vi "Read Gates From Registry.vi"(7 "Micropulse No.":i32, 8 "error in (no error)":errorcluster, 11 "Test No.":u32) -> (0 "error out":errorcluster, 1 "Multi Gate Inspection":T3 {"Gate 4"."Max # Peaks" max=64000 step=100; "Gate 4"."Threshold" min=10 max=4095 step=10; "Gate 4"."Length (us)" min=0.0 max=96000.0 step=100.0; "Gate 4"."Start (us)" min=0.0 max=64000.0 step=100.0; "Gate 3"."Max # Peaks" max=64000 step=100; "Gate 3"."Threshold" min=10 max=4095 step=10; "Gate 3"."Length (us)" min=0.0 max=96000.0 step=100.0; "Gate 3"."Start (us)" min=0.0 max=64000.0 step=100.0; "Gate 2"."Max # Peaks" max=64000 step=100; "Gate 2"."Threshold" min=10 max=4095 step=10; "Gate 2"."Length (us)" min=0.0 max=96000.0 step=100.0; "Gate 2"."Start (us)" min=0.0 max=64000.0 step=100.0; "Gate 1"."Max # Peaks" max=64000 step=100; "Gate 1"."Threshold" min=10 max=4095 step=10; "Gate 1"."Length (us)" min=0.0 max=96000.0 step=100.0; "Gate 1"."Start (us)" min=0.0 max=64000.0 step=100.0}, 2 "Echo Gate Parameters":T2={"Start (us)"=0.0, "Length (us)"=0.0, "Threshold"=10} {"Threshold" min=10 max=4095 step=10; "Length (us)" min=0.0 max=96000.0 step=100.0; "Start (us)" min=0.0 max=64000.0 step=100.0}, 3 "Echo Gate Mode":T1)   [LabVIEW 2015]
uses:
  <instrlib>/Micropulse/Public/Data/Datatypes/MP - multi-gate inspection.ctl
  <instrlib>/Micropulse/Public/Data/Datatypes/MP - multigate inspection gate parameters.ctl
  <instrlib>/Micropulse/Public/Data/Datatypes/MP - hysteresis level.ctl
  <instrlib>/Micropulse/Public/Data/Datatypes/MP - multigate mode.ctl
  <instrlib>/Micropulse/Public/Data/Datatypes/MP - echo gate parameters.ctl
  <instrlib>/Micropulse/Public/Data/Datatypes/MP - echo gate mode.ctl
  <instrlib>/Micropulse/Micropulse.lvlib
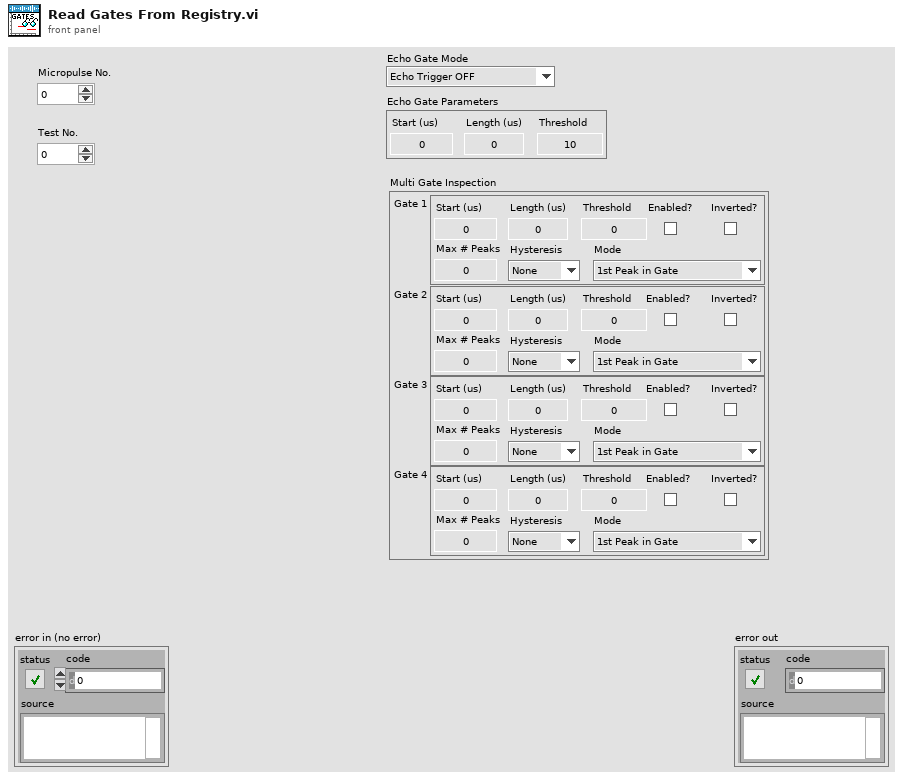
[diagram p1: front panel]
types:
  T1 = typedef "Micropulse.lvlib/MP - echo gate mode.ctl" = enum16{"Echo Trigger OFF", "Echo Gate Display Mode", "Echo Trigger ON", "Multi Gate or FMC Mode", "Reserved", "PA - Echo Trigger ON"}
  T2 = typedef "MP - echo gate parameters.ctl" = cluster{"Start (us)":dbl, "Length (us)":dbl, "Threshold":u16}
  T3 = typedef "MP - multi-gate inspection.ctl" = cluster{"Gate 1":T4, "Gate 2":T4, "Gate 3":T4, "Gate 4":T4}
  T4 = typedef "Micropulse.lvlib/MP - multigate inspection gate parameters.ctl" = cluster{"Start (us)":dbl, "Length (us)":dbl, "Threshold":u16, "Enabled?":bool, "Max # Peaks":u16, "Hysteresis":T5, "Mode":T6, "Inverted?":bool}
  T5 = typedef "Micropulse.lvlib/MP - hysteresis level.ctl" = enum16{"None", "3dB", "6dB", "9dB", "12dB"}
  T6 = typedef "Micropulse.lvlib/MP - multigate mode.ctl" = enum16{"1st Peak in Gate", "Largest Peak In Gate", "All Peaks In Gate", "1st Threshold Crossing"}
  T7 = typedef "Micropulse.lvlib/MP-Registry Data-Cluster.ctl" = cluster{"Instrument Type":T8, "Serial #":u64, "Sample Frequency":T9, "dt (us)":dbl, "DOF":T10, "Material Velocity":dbl, "Asynch Reads":T11, "NUM of Tests":u16, "Gates":T12[], "CMD LUT":variant, "Command List":string}
  T8 = typedef "Micropulse.lvlib/MP - instrument type.ctl" = enum16{"MicroPulse 5", "MicroPulse LT1", "MicroPulse LT2", "MicroPulse LTPA", "MPLT", "MicroPulse 6", "<MicroPulse>", "Simulated Data"}
  T9 = typedef "Micropulse.lvlib/MP - sample frequency.ctl" = enum16{"Use Default", "200MHz (LT2 only)", "100MHz", "50MHz", "25MHz", "10MHz"}
  T10 = typedef "Micropulse.lvlib/MP - data output format.ctl" = enum16{"", "8-bit Mode", "10-bit Mode", "12-bit Mode", "16-bit Mode", "8-bit Log Mode", "12-bit Packed Mode"}
  T11 = typedef "Micropulse.lvlib/MP - asynch read mode.ctl" = enum16{"Disabled", "Enabled"}
  T12 = typedef "Micropulse.lvlib/MP - Registry Gates.ctl" = cluster{"Display Gate":T13, "ETM Mode":T1, "Echo Gate":T2, "Insp Gates":T4[]}
  T13 = typedef "MP - display gate.ctl" = cluster{"Start":dbl, "Length":dbl}
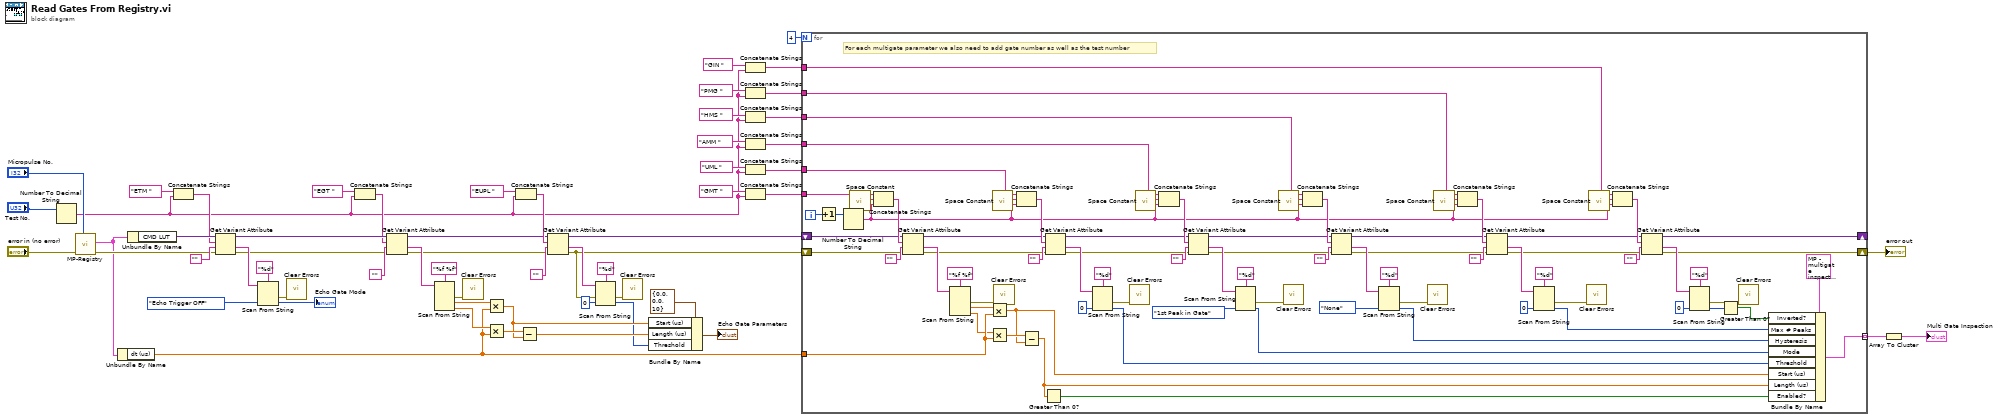
[diagram p0: block diagram]
diagram:
  n1 = Number To Decimal String(number="Test No.") -> (decimal integer string=w12:string)  [unwired: 1 in]
  n2 = call <instrlib>:"MP-Registry.vi"("Micropulse # In"="Micropulse No.", "error in (no error)"="error in (no error)") -> ("error out"=w54:errorcluster, "Micropulse Data"=w35:T7)  [unwired: 6 in, 2 out]
  n3 = Unbundle By Name(w35) -> ("dt (us)"=w20:dbl)
  n4 = Unbundle By Name(w35) -> ("CMD LUT"=w57:variant)
  n5 = Concatenate Strings("ETM " ("name"), w12) -> (w46:string)
  n6 = Get Variant Attribute(Variant=w57, name=w46, default value (empty Variant)="", error in=w54) -> (duplicate Variant=w49:variant, value=w53:string, error out=w4:errorcluster)  [unwired: 1 out]
  n7 = Scan From String(format string="%d", input string=w53, default 1=MP_-_echo_gate_mode."Echo Trigger OFF" ("Echo Gate Mode")) -> (error out=w2:errorcluster, output 1=→"Echo Gate Mode":T1)  [unwired: 2 in, 2 out]
  n8 = call <vilib>:"Clear Errors.vi"("error in (no error)"=w2) -> ()  [unwired: 5 in, 2 out]
  n9 = Concatenate Strings("EGT " ("name"), w12) -> (w44:string)
  n10 = Get Variant Attribute(Variant=w49, name=w44, default value (empty Variant)="", error in=w4) -> (duplicate Variant=w27:variant, value=w42:string, error out=w5:errorcluster)  [unwired: 1 out]
  n11 = Scan From String(format string="%f %f", input string=w42) -> (error out=w1:errorcluster, output 1=w34:dbl, output 2=w33:dbl)  [unwired: 4 in, 2 out]
  n12 = call <vilib>:"Clear Errors.vi"("error in (no error)"=w1) -> ()  [unwired: 5 in, 2 out]
  n13 = Multiply(x=w34, y=w20) -> (x*y=w29:dbl)
  n14 = Multiply(x=w33, y=w20) -> (x*y=w32:dbl)
  n15 = Concatenate Strings("EUPL " ("name"), w12) -> (w39:string)
  n16 = Subtract(x=w32, y=w29) -> (x-y=w30:dbl)
  n17 = Get Variant Attribute(Variant=w27, name=w39, default value (empty Variant)="", error in=w5) -> (duplicate Variant=w22:variant, value=w41:string, error out=w3:errorcluster)  [unwired: 1 out]
  n18 = Scan From String(format string="%d", input string=w41, error in=w3, default 1=u16 0 ("default value 1")) -> (error out=w21:errorcluster, output 1=w28:u16)  [unwired: 1 in, 2 out]
  n19 = call <vilib>:"Clear Errors.vi"("error in (no error)"=w21) -> ()  [unwired: 5 in, 2 out]
  n20 = Bundle By Name(cluster=T2 {"Start (us)"=0.0, "Length (us)"=0.0, "Threshold"=10} ("Echo Gate Parameters"), "Start (us)"=w29, "Length (us)"=w30, "Threshold"=w28) -> (→"Echo Gate Parameters":T2)
  n21 = Concatenate Strings("GIN " ("name"), w12) -> (w9:string)
  n22 = Concatenate Strings("PMG " ("name"), w12) -> (w10:string)
  n23 = Concatenate Strings("HMS " ("name"), w12) -> (w11:string)
  n24 = Concatenate Strings("AMM " ("name"), w12) -> (w16:string)
  n25 = Concatenate Strings("UML " ("name"), w12) -> (w18:string)
  n26 = Concatenate Strings("GMT " ("name"), w12) -> (w24:string)
  n27 = for {
    N: 4 -> [_]
    tunnel: w24 -> [w137]
    shift-right: [w88] -> _
    shift-left: w22 -> [w130]
    shift-right: [w69] -> w8
    shift-left: w3 -> [w129]
    tunnel: w20 -> [w126]
    tunnel: w18 -> [w119]
    tunnel: w16 -> [w111]
    tunnel: w11 -> [w86]
    tunnel: w10 -> [w85]
    tunnel: w9 -> [w84]
    tunnel: [w73] -> w7 mode=indexing
    i -> [w133]
    # "For each multigate parameter we also need to add gate number as well as the test number"
    n28 = Increment(x=w133) -> (x+1=w132:i32)
    n29 = Number To Decimal String(number=w132) -> (decimal integer string=w72:string)  [unwired: 1 in]
    n30 = call <vilib>:"Space Constant.vi"() -> ("String"=w131:string)
    n31 = Concatenate Strings(w137, w131, w72) -> (w134:string)
    n32 = Get Variant Attribute(Variant=w130, name=w134, default value (empty Variant)="", error in=w129) -> (duplicate Variant=w118:variant, value=w135:string, error out=w71:errorcluster)  [unwired: 1 out]
    n33 = Scan From String(format string="%f %f", input string=w135) -> (error out=w70:errorcluster, output 1=w127:dbl, output 2=w125:dbl)  [unwired: 4 in, 2 out]
    n34 = Multiply(x=w127, y=w126) -> (x*y=w74:dbl)
    n35 = Multiply(x=w125, y=w126) -> (x*y=w128:dbl)
    n36 = call <vilib>:"Space Constant.vi"() -> ("String"=w124:string)
    n37 = call <vilib>:"Clear Errors.vi"("error in (no error)"=w70) -> ()  [unwired: 5 in, 2 out]
    n38 = Concatenate Strings(w119, w124, w72) -> (w120:string)
    n39 = Subtract(x=w128, y=w74) -> (x-y=w75:dbl)
    n40 = Greater Than 0?(x=w75) -> (x > 0?=w76:bool)
    n41 = Get Variant Attribute(Variant=w118, name=w120, default value (empty Variant)="", error in=w71) -> (duplicate Variant=w109:variant, value=w123:string, error out=w61:errorcluster)  [unwired: 1 out]
    n42 = Scan From String(format string="%d", input string=w123, default 1=u16 0 ("default value 1")) -> (error out=w60:errorcluster, output 1=w77:u16)  [unwired: 2 in, 2 out]
    n43 = call <vilib>:"Clear Errors.vi"("error in (no error)"=w60) -> ()  [unwired: 5 in, 2 out]
    n44 = call <vilib>:"Space Constant.vi"() -> ("String"=w112:string)
    n45 = Concatenate Strings(w111, w112, w72) -> (w116:string)
    n46 = Get Variant Attribute(Variant=w109, name=w116, default value (empty Variant)="", error in=w61) -> (duplicate Variant=w91:variant, value=w113:string, error out=w63:errorcluster)  [unwired: 1 out]
    n47 = Scan From String(format string="%d", input string=w113, default 1=MP_-_multigate_mode."1st Peak in Gate" ("Value")) -> (error out=w62:errorcluster, output 1=w78:T6)  [unwired: 2 in, 2 out]
    n48 = call <vilib>:"Space Constant.vi"() -> ("String"=w104:string)
    n49 = call <vilib>:"Clear Errors.vi"("error in (no error)"=w62) -> ()  [unwired: 5 in, 2 out]
    n50 = Concatenate Strings(w86, w104, w72) -> (w108:string)
    n51 = Get Variant Attribute(Variant=w91, name=w108, default value (empty Variant)="", error in=w63) -> (duplicate Variant=w90:variant, value=w105:string, error out=w65:errorcluster)  [unwired: 1 out]
    n52 = Scan From String(format string="%d", input string=w105, default 1=MP_-_hysteresis_level."None" ("Value")) -> (error out=w64:errorcluster, output 1=w79:T5)  [unwired: 2 in, 2 out]
    n53 = call <vilib>:"Clear Errors.vi"("error in (no error)"=w64) -> ()  [unwired: 5 in, 2 out]
    n54 = call <vilib>:"Space Constant.vi"() -> ("String"=w103:string)
    n55 = Concatenate Strings(w85, w103, w72) -> (w99:string)
    n56 = Get Variant Attribute(Variant=w90, name=w99, default value (empty Variant)="", error in=w65) -> (duplicate Variant=w89:variant, value=w102:string, error out=w67:errorcluster)  [unwired: 1 out]
    n57 = Scan From String(format string="%d", input string=w102, default 1=u16 0 ("default value 1")) -> (error out=w66:errorcluster, output 1=w80:u16)  [unwired: 2 in, 2 out]
    n58 = call <vilib>:"Clear Errors.vi"("error in (no error)"=w66) -> ()  [unwired: 5 in, 2 out]
    n59 = call <vilib>:"Space Constant.vi"() -> ("String"=w92:string)
    n60 = Concatenate Strings(w84, w92, w72) -> (w96:string)
    n61 = Get Variant Attribute(Variant=w89, name=w96, default value (empty Variant)="", error in=w67) -> (duplicate Variant=w88:variant, value=w93:string, error out=w69:errorcluster)  [unwired: 1 out]
    n62 = Scan From String(format string="%d", input string=w93, default 1=u16 0 ("default value 1")) -> (error out=w68:errorcluster, output 1=w82:u16)  [unwired: 2 in, 2 out]
    n63 = Greater Than 0?(x=w82) -> (x > 0?=w81:bool)
    n64 = call <vilib>:"Clear Errors.vi"("error in (no error)"=w68) -> ()  [unwired: 5 in, 2 out]
    n65 = Bundle By Name(cluster=T4 {"Start (us)"=0.0, "Length (us)"=0.0, "Threshold"=0, "Enabled?"=FALSE, "Max # Peaks"=0, "Hysteresis"=enum."None", "Mode"=enum."1st Peak in Gate", "Inverted?"=FALSE} ("Gate 1"), "Inverted?"=w81, "Max # Peaks"=w80, "Hysteresis"=w79, "Mode"=w78, "Threshold"=w77, "Start (us)"=w74, "Length (us)"=w75, "Enabled?"=w76) -> (w73:T4)
  }
  "error out" <- w8
  n66 = Array To Cluster(array=w7) -> (cluster=→"Multi Gate Inspection":cluster{"[0]":T4, "[1]":T4, "[2]":T4, "[3]":T4})
